vi "Thermal Chamber Controller_DQMH_Action Update Heater State-setup.vi"(11 "test case ID":string) -> (3 "Heater State":T1)   [LabVIEW 2018]
doc: "The setup VI should be executed before the VI under test in the harness VI. In this VI you can prepare the environment and the inputs of the VI under test.\n\nSee the Help Document for more information. (<b>Help</b> > <b>IncQuery Labs</b> > <b>InstaCoverage</b> > <b>InstaCoverage Help...</b>)"
uses:
  Libraries/Thermal Chamber Controller_DQMH/Heater State--enum.ctl
  Libraries/Thermal Chamber Controller_DQMH/Thermal Chamber Controller_DQMH.lvlib
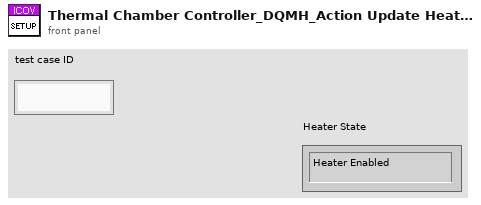
[diagram p1: front panel]
types:
  T1 = typedef "Thermal Chamber Controller_DQMH.lvlib/Heater State--enum.ctl" = enum16{"Heater Enabled", "Heater Disabled"}
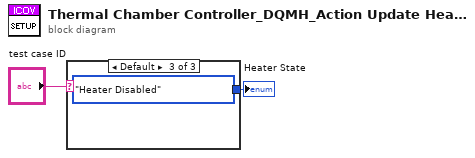
[diagram p0: block diagram]
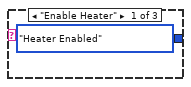
[diagram p2: hidden frame]
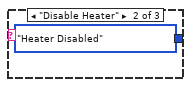
[diagram p3: hidden frame]
diagram:
  n1 = case shown="Default" "test case ID" {
    tunnel: [Heater_State--enum."Heater Enabled" ("Heater State Result") Heater_State--enum."Heater Disabled" ("Heater State Result") Heater_State--enum."Heater Disabled" ("Heater State Result")] -> w2
    frame "Enable Heater" {
    }
    frame "Disable Heater" {
    }
    frame Default {
    }
  }
  "Heater State" <- w2
